vi "NoisySine.vi"() -> ()   [LabVIEW 2013]
panel:
  out "XY Graph":cluster{dbl[], dbl[]}(graph)
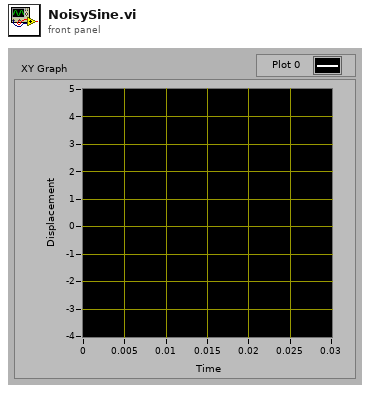
[diagram p1: front panel]
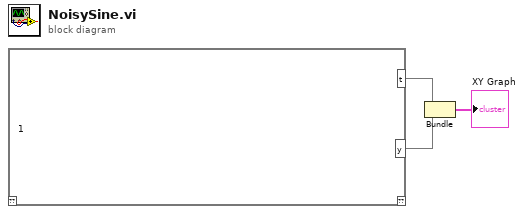
[diagram p0: block diagram]
diagram:
  n1 = mathscript code="1"() -> ("t"=w3, "y"=w2)  [unwired: 1 in, 1 out]
  n2 = Bundle("t"=w3, "y"=w2) -> (→"XY Graph":cluster{"t":void, "y":void})  [unwired: 1 in]
